vi "Replace Diagram Contents.vi"(8 "error in (no error)":errorcluster, 10 "Template VI":path, 11 "Target VI":refnum<vi>) -> (0 "error out":errorcluster, 3 "dup Target VI":refnum<vi>)   [LabVIEW 2020, in "Message Rescripter.lvlib"]
uses:
  Message Rescripter.lvlib
  <vilib>/Utility/traverseref.llb/VI Scripting - Traverse.lvlib
  <vilib>/Utility/traverseref.llb/TRef TravTarget.ctl
  <vilib>/Utility/miscctls.llb/LVPointTypeDef.ctl
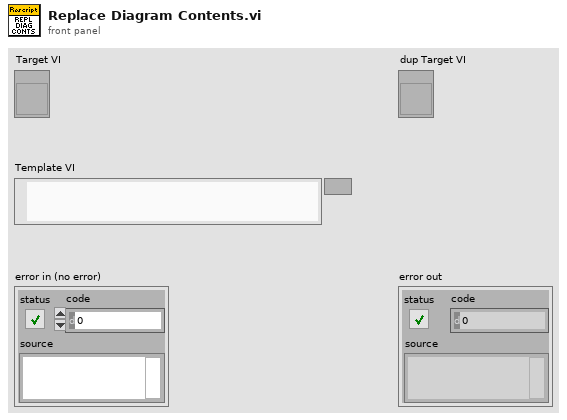
[diagram p1: front panel]
types:
  T1 = typedef "LVPointTypeDef.ctl" = cluster{"Horizontal":i16, "Vertical":i16}
  T2 = typedef "TRef TravTarget.ctl" = enum16{"FP", "BD", "Other"}
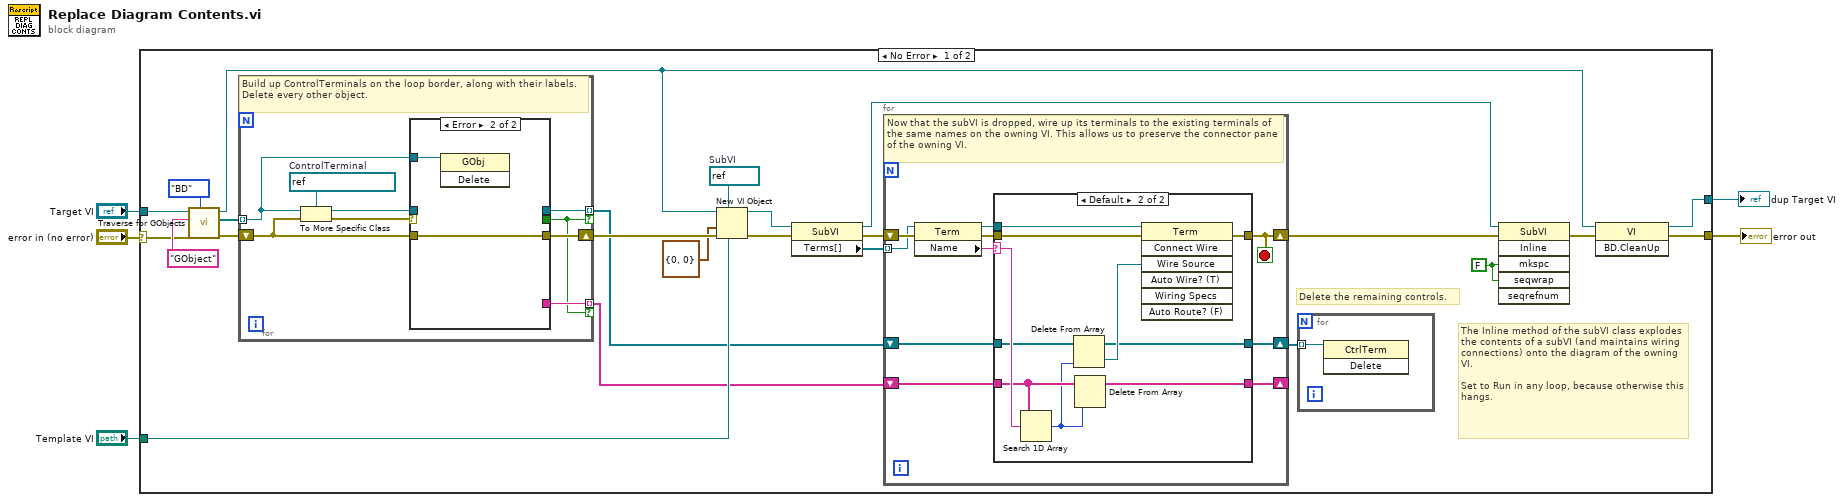
[diagram p0: block diagram]
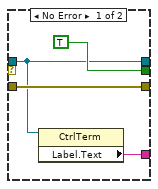
[diagram p3: hidden frame]
diagram:
  n1 = case shown="No Error" "error in (no error)" {
    selector: "error in (no error)" -> [w6 w70]
    tunnel: "Template VI" -> [w25 _]
    tunnel: [w24 w70] -> w4
    tunnel: "Target VI" -> [w23 w69]
    tunnel: [w9 w69] -> w2
    frame No Error {
      w10 = FALSE
      w19 = refnum<vi> refnum  # SubVI
      # "The Inline method of the subVI class explodes the contents of a subVI (and maintains wiring connections) onto the diagram of the owning VI.\n\nSet to Run in any loop, because otherwise this hangs."
      # "Delete the remaining controls."
      n2 = call <vilib>:"Traverse for GObjects.vi"("Traverse Target"=TRef_TravTarget."BD", "error in (no error)"=w6, "Class Name"="GObject", "VI Refnum"=w23) -> ("error out"=w27:errorcluster, "References"=w26:refnum<vi>[], "dup VI Refnum"=w8:refnum<vi>)  [unwired: 4 in, 1 out]
      n3 = for {
        tunnel: w26 -> [w58] mode=indexing
        tunnel: [w59] -> w21 mode=indexing if=w54
        shift-right: [w56] -> w22
        shift-left: w27 -> [w57]
        tunnel: [w55] -> w20 mode=indexing if=w54
        w62 = refnum<vi> refnum  # ControlTerminal
        # "Build up ControlTerminals on the loop border, along with their labels. Delete every other object."
        n4 = To More Specific Class(target class=w62, reference=w58, error in=w57) -> (specific class reference=w60:refnum<vi>, error out=w61:errorcluster)
        n5 = case shown="Error" w61 {
          tunnel: w60 -> [w64 _]
          tunnel: [w64 _] -> w59
          tunnel: [TRUE _] -> w54
          tunnel: w58 -> [_ w68]
          tunnel: w57 -> [w65 w67]
          tunnel: [w65 w67] -> w56
          tunnel: [w63 _] -> w55
          frame No Error {
            n6 = property class="CtrlTerm"(reference=w64) -> ("Label.Text"=w63:string)  [unwired: 1 in, 2 out]
          }
          frame Error {
            n7 = invoke class="GObj" method="Delete"(reference=w68) -> ()  [unwired: 2 in, 3 out]
          }
        }
      }
      n8 = New VI Object(vi object class=w19, owner refnum=w8, position/next to=T1 {"Horizontal"=0, "Vertical"=0} ("location"), 6:w25, 8:w22) -> (object refnum=w16:refnum<vi>, 0:w17:errorcluster)  [unwired: 3 in]
      n9 = property class="SubVI"(reference=w16, error in=w17) -> (reference out=w13:refnum<vi>, error out=w15:errorcluster, "Terms[]"=w14:refnum<vi>[])
      n10 = for {
        shift-right: [w33] -> w7
        shift-left: w15 -> [w40]
        tunnel: w14 -> [w39] mode=indexing
        shift-right: [w32] -> w12
        shift-left: w21 -> [w36]
        shift-right: [w31] -> _
        shift-left: w20 -> [w38]
        stop <- w33 stop-if-true
        # "Now that the subVI is dropped, wire up its terminals to the existing terminals of the same names on the owning VI. This allows us to preserve the connector pane of the owning VI."
        n11 = property class="Term"(reference=w39, error in=w40) -> (reference out=w34:refnum<vi>, error out=w35:errorcluster, "Name"=w37:string)
        n12 = case shown="Default" w37 {
          selector: w37 -> [_ w53]
          tunnel: w38 -> [w41 w46]
          tunnel: w36 -> [w42 w52]
          tunnel: w35 -> [w43 w51]
          tunnel: w34 -> [_ w50]
          tunnel: [w43 w49] -> w33
          tunnel: [w42 w47] -> w32
          tunnel: [w41 w44] -> w31
          frame "" {
          }
          frame Default {
            n13 = Search 1D Array(1D array=w46, element=w53) -> (index of element=w45:i32)  [unwired: 1 in]
            n14 = Delete From Array(array=w52, index=w45) -> (deleted portion=w48:refnum<vi>, array with subset deleted=w47:refnum<vi>[])  [unwired: 1 in]
            n15 = Delete From Array(array=w46, index=w45) -> (array with subset deleted=w44:string[])  [unwired: 1 in, 1 out]
            n16 = invoke class="Term" method="Connect Wire"(reference=w50, error in=w51, "Wire Source"=w48) -> (error out=w49:errorcluster)  [unwired: 4 in, 6 out]
          }
        }
      }
      n17 = for {
        tunnel: w12 -> [w30] mode=indexing
        n18 = invoke class="CtrlTerm" method="Delete"(reference=w30) -> ()  [unwired: 2 in, 3 out]
      }
      n19 = invoke class="SubVI" method="Inline"(reference=w13, error in=w7, "mkspc"=w10, "seqwrap"=w10) -> (error out=w11:errorcluster)  [unwired: 2 in, 5 out]
      n20 = invoke class="VI" method="BD.CleanUp"(reference=w8, error in=w11) -> (reference out=w9:refnum<vi>, error out=w24:errorcluster)  [unwired: 1 in, 1 out]
    }
    frame Error {
    }
  }
  "error out" <- w4
  "dup Target VI" <- w2
